vi "speak.vi"(8 "error in (no error)":errorcluster, 11 "Cat in":refnum<class "Cat.lvclass">) -> (0 "error out":errorcluster, 3 "Cat out":refnum<class "Cat.lvclass">)   [LabVIEW 2021, in "Cat.lvclass"]
uses:
  Cat.lvclass
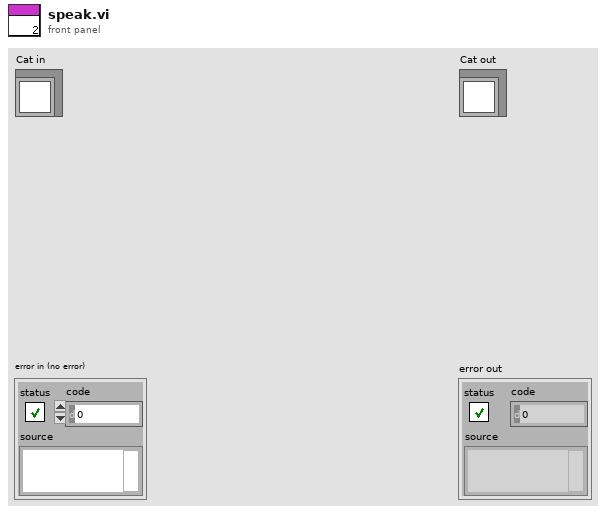
[diagram p1: front panel]
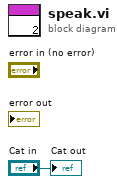
[diagram p0: block diagram]
diagram:
  "Cat out" <- "Cat in"
